vi "ReadConfigFile.vi"(11 "AppGUID":string[](array[string])=["{F4DE796F-D708-47C6-9A47-E097E595CC62}", "{5076E98B-8725-47A3-AC71-540803FA6786}", "{98ED115E-F3D7-42E1-95EC-D5A701E8606C}", "{41638F72-A3B1-4571-9D24-805CD0A5C916}", "{DFCDA2DF-D74A-2A0B-78D2-1E43916DC130}", "{5C2805AD-F36C-6735-F3D2-1E34979F1738}", "{D3623530-08AF-4E67-8152-0FF6253B2CCF}", "{2DFD17FF-624E-431C-8EC7-7EA8C60D5693}", "{E531E5B0-C41D-43CC-A40E-D3AD13AED942}", "{7F992673-D125-475F-9434-B27C83393E0F}"]) -> (3 "ImageName":string[](array[string]))   [LabVIEW 2016]
uses:
  <vilib>/Utility/config.llb/Read Key (String).vi
  <vilib>/Utility/config.llb/NI_LVConfig.lvlib
panel:
  out "appended path":path
  out "found?":bool
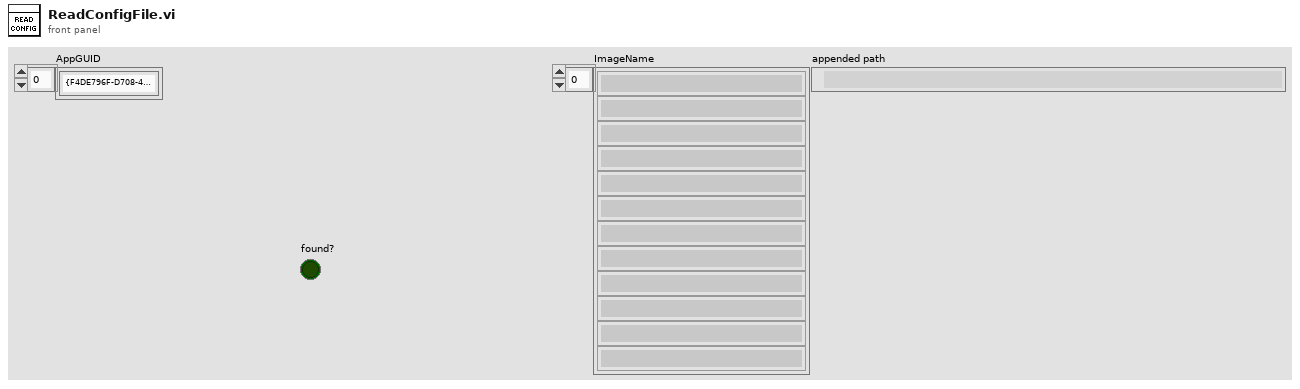
[diagram p1: front panel]
types:
  T1 = typedef "NI_LVConfig.lvlib/Config Data RefNum.ctl" = refnum<k1>
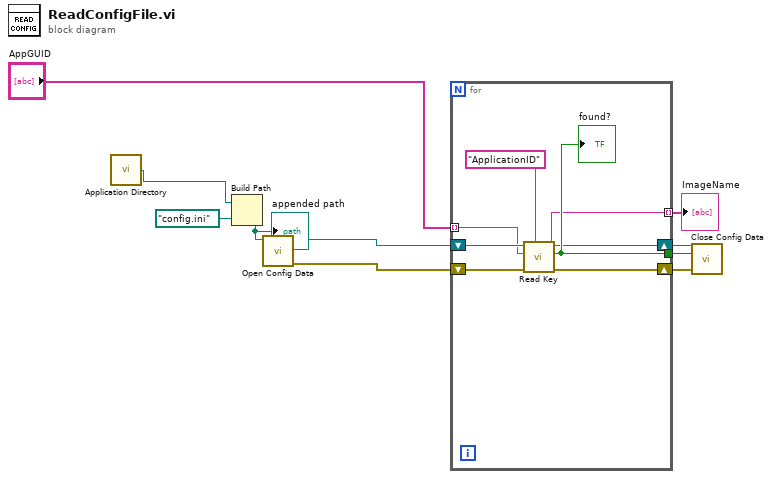
[diagram p0: block diagram]
diagram:
  n1 = call <vilib>:"Application Directory.vi"() -> ("Application Directory"=w1:path)
  n2 = Build Path(base path=w1, name or relative path=path "config.ini" ("configuration file path")) -> (appended path=w3:path)
  "appended path" <- w3
  n3 = call <vilib>:"Open Config Data.vi"("configuration file path"=w3) -> ("error out"=w10:errorcluster, "refnum"=w9:T1)  [unwired: 8 in, 1 out]
  n4 = for {
    tunnel: [w15] -> w7
    tunnel: [w12] -> w4 mode=indexing
    shift-right: [w16] -> w8
    shift-left: w10 -> [w18]
    shift-right: [w14] -> w6
    shift-left: w9 -> [w17]
    tunnel: "AppGUID" -> [w11] mode=indexing
    n5 = call-poly <vilib>:"Read Key.vi"("section"="ApplicationID", "error in (no error)"=w18, "key"=w11, "refnum"=w17) -> ("error out"=w16:errorcluster, "value"=w12:string, "found?"=w15:bool, "refnum out"=w14:T1)  [unwired: 4 in]
    "found?" <- w15
  }
  "ImageName" <- w4
  n6 = call <vilib>:"Close Config Data.vi"("error in (no error)"=w8, "write file if changed (T)"=w7, "refnum"=w6) -> ()  [unwired: 7 in, 2 out]
